vi "To Binary.vi"(6 "byte order":T1(ring), 8 "error in (no error)":errorcluster, 11 "Double Float in":refnum<class "Abs_I16 Integer 1D.lvclass">) -> (0 "error out":errorcluster, 2 "Binary":string, 3 "Double Float out":refnum<class "Abs_I16 Integer 1D.lvclass">)   [LabVIEW 2021, in "Abs_I16 Integer 1D.lvclass"]
uses:
  Abs_I16 Integer 1D.lvclass
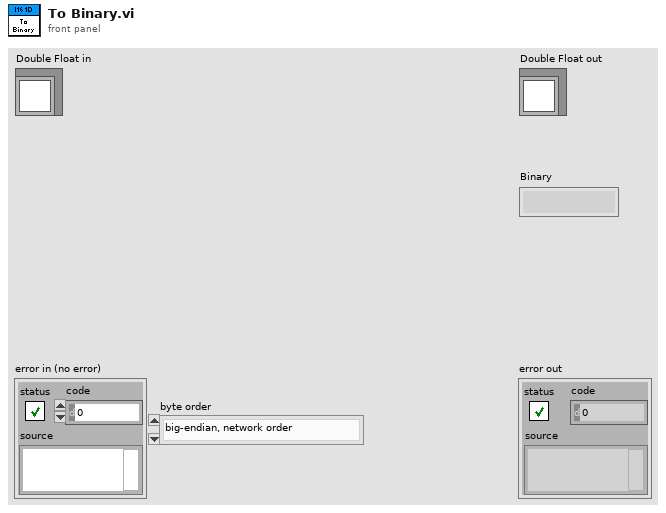
[diagram p1: front panel]
types:
  T1 = enum16{"big-endian, network order", "native, host order", "little-endian"}
  T2 = typedef "Abs_I16 Integer 1D.lvclass/Type.ctl" = i16[]
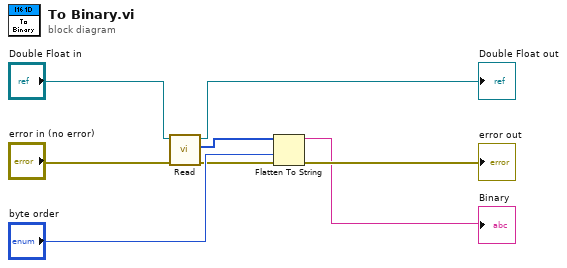
[diagram p0: block diagram]
diagram:
  n1 = call-dynamic "Read.vi"("error in (no error)"="error in (no error)", "Double Float.lvclass_340760 in"="Double Float in") -> ("error out"=w1:errorcluster, "Value"=w2:T2, "Double Float.lvclass_340760 out"=→"Double Float out":refnum<class "Abs_I16 Integer 1D.lvclass">)  [unwired: 7 in]
  n2 = Flatten To String(anything=w2, byte order (0:big-endian, network order)="byte order", error in (no error)=w1) -> (data string=→"Binary":string, error out=→"error out":errorcluster)  [unwired: 1 in, 1 out]
